vi "example batch nowait.vi"() -> ()   [LabVIEW 2013]
uses:
  result/result.lvclass
  standard action/wait action/wait action.lvclass
  standard tasks/batch task/reporting type.ctl
  result/result.lvclass/result.ctl
  result/get data.vi
  result/get error.vi
  result/get generating action.vi
  result/get owning task.vi
  result/get subresults.vi
  dispatcher/thread pool.lvclass
  standard reporters/event reporter/event reporter.lvclass
  standard tasks/batch task/batch task.lvclass
panel:
  out "return times":u32[](array[numeric])
  out "iteration":i32
  out "result":refnum<class "result.lvclass">[](array[class])
  out "accessors:subresults":refnum<class "result.lvclass">[][](array[class])
  out "owning task":string[](array[string])
  out "actions":string[](array[string])
  out "Array 2":errorcluster[](array[cluster])
  out "Array":variant[](array[variant])
  out "Time":u32
  out "error out":errorcluster
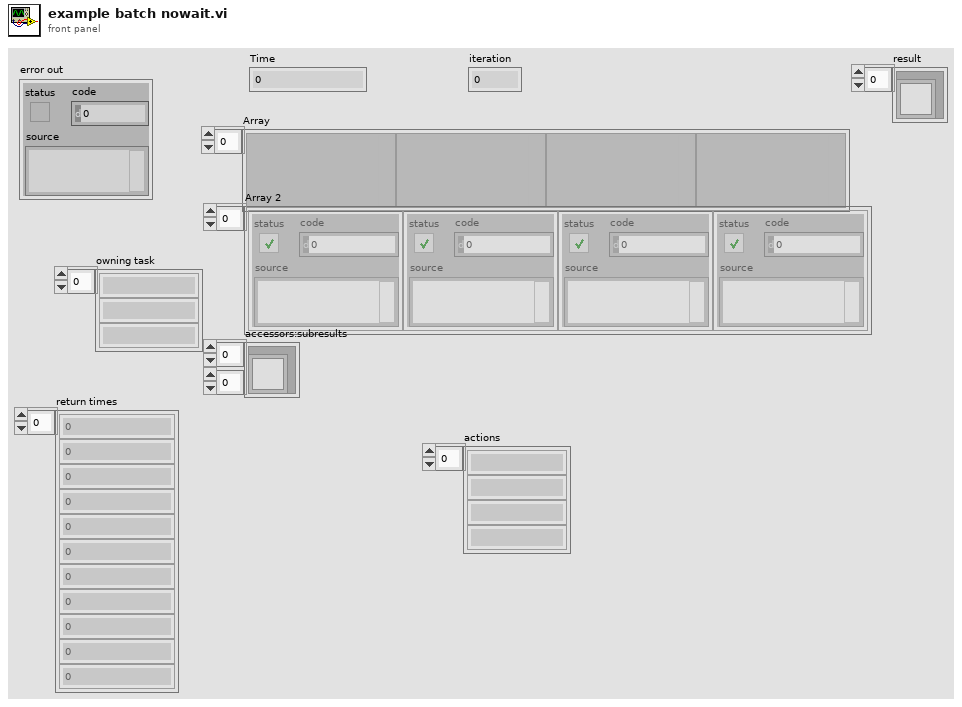
[diagram p1: front panel]
types:
  T1 = typedef "batch task.lvclass/reporting type.ctl" = enum16{"return immediately", "wait on all"}
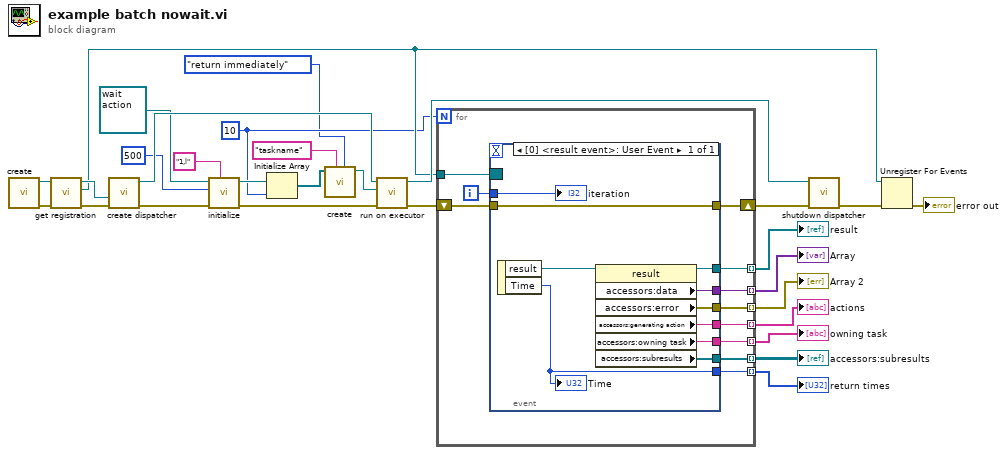
[diagram p0: block diagram]
diagram:
  w9 = 10 ("dimension size")
  n1 = call "create.vi"() -> ("error out"=w24:errorcluster, "event reporter out"=w25:refnum<class "event reporter.lvclass">)  [unwired: 10 in]
  n2 = call "get registration.vi"("error in"=w24, "event reporter in"=w25) -> ("error out"=w22:errorcluster, "result registration"=w10:refnum<event-registration>, "event reporter out"=w23:refnum<class "event reporter.lvclass">)  [unwired: 7 in]
  n3 = call "create dispatcher.vi"("error in"=w22, "default reporter"=w23) -> ("error out"=w27:errorcluster, "dispatcher"=w29:refnum<data-value>)  [unwired: 8 in]
  n4 = call-dynamic "initialize.vi"("action name"="1,l", "error in"=w27, "parameters"=500, "action in"=refnum<class "wait action.lvclass"> refnum ("wait action.lvclass")) -> ("error out"=w15:errorcluster, "action out"=w16:refnum<class "wait action.lvclass">)  [unwired: 6 in]
  n5 = Initialize Array(w16, w9) -> (w13:refnum<class "wait action.lvclass">[])
  n6 = call "create.vi"("reporting type"=reporting_type."return immediately", "ID"="taskname", "actions"=w13) -> ("batch task out"=w12:refnum<class "batch task.lvclass">)  [unwired: 8 in]
  n7 = call "run on executor.vi"("error in"=w15, "task"=w12, "dispatcher"=w29) -> ("error out"=w17:errorcluster, "dispatcher out"=w21:refnum<data-value>)  [unwired: 7 in]
  n8 = for {
    N: w9 -> [_]
    tunnel: w10 -> [w40]
    shift-right: [w39] -> w18
    shift-left: w17 -> [w38]
    tunnel: [w37] -> w8 mode=indexing
    tunnel: [w36] -> w7 mode=indexing
    tunnel: [w35] -> w6 mode=indexing
    tunnel: [w34] -> w5 mode=indexing
    tunnel: [w33] -> w4 mode=indexing
    tunnel: [w32] -> w3 mode=indexing
    tunnel: [w30] -> w2 mode=indexing
    i -> [w31]
    n9 = event shown="[0] <result event>: User Event" {
      selector: w40 -> [_]
      dyn-events: _ -> [_]
      timeout: _ -> [_]
      tunnel: [w50] -> w39
      tunnel: w38 -> [w50]
      tunnel: [w48] -> w37
      tunnel: [w47] -> w36
      tunnel: [w46] -> w35
      tunnel: [w45] -> w34
      tunnel: [w44] -> w33
      tunnel: [w43] -> w32
      tunnel: w31 -> [w42]
      tunnel: [w41] -> w30
      event User Event {
        n10 = event-data() -> ("result"=w49:refnum<class "result.lvclass">, "Time"=w41:u32)  [unwired: 1 in]
        "Time" <- w41
        n11 = property class="result"(reference=w49) -> (reference out=w43:refnum<class "result.lvclass">, "accessors:data"=w48:variant, "accessors:error"=w47:errorcluster, "accessors:generating action"=w46:string, "accessors:owning task"=w45:string, "accessors:subresults"=w44:refnum<class "result.lvclass">[])  [unwired: 1 in, 1 out]
        "iteration" <- w42
      }
    }
  }
  "Array" <- w8
  "Array 2" <- w7
  "actions" <- w6
  "owning task" <- w5
  "accessors:subresults" <- w4
  "result" <- w3
  "return times" <- w2
  n12 = call "shutdown dispatcher.vi"("error in"=w18, "dispatcher"=w21) -> ("error out"=w20:errorcluster)  [unwired: 9 in]
  n13 = Unregister For Events(event registration refnum=w10, error in=w20) -> (error out=→"error out":errorcluster)
